vi "NGwrite_imp.vi"(0 "Unresolved URL":string, 1 "buffer value limit":u32=1, 5 "Cached URL":string, 7 "Data":variant, 9 "buffer size limit":u32=4294967295, 11 "error in":errorcluster) -> (15 "error out":errorcluster)   [LabVIEW 2017]
uses:
  nitaglv.dll
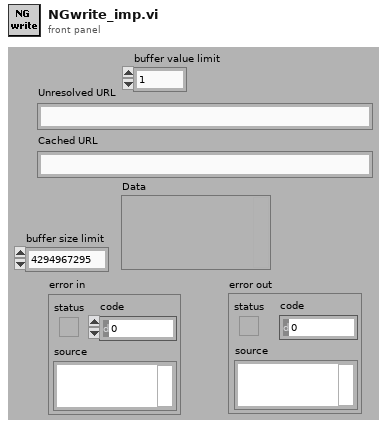
[diagram p1: front panel]
types:
  T1 = cluster{"timestamp":bool, "write":bool, "buffer size limit":u32, "buffer value limit":u32, "delta filter":bool}
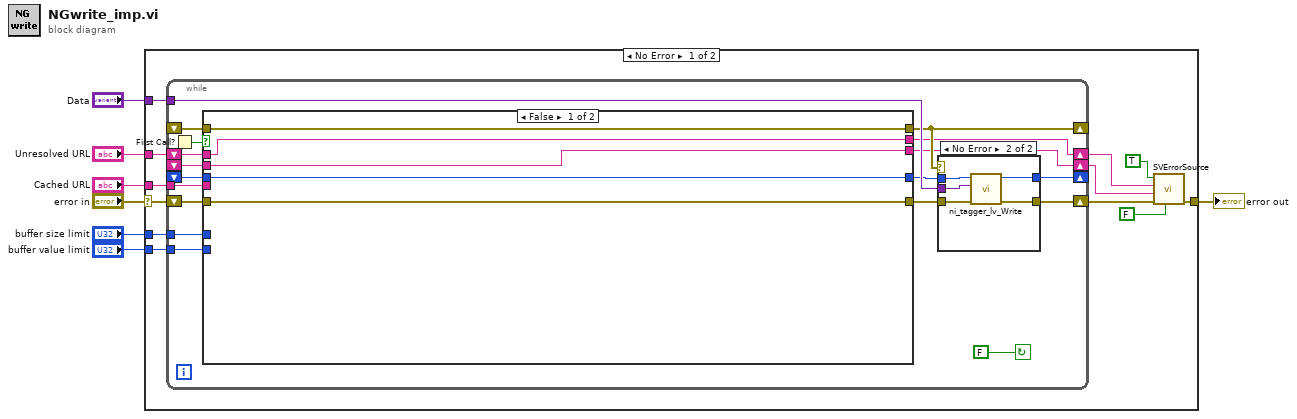
[diagram p0: block diagram]
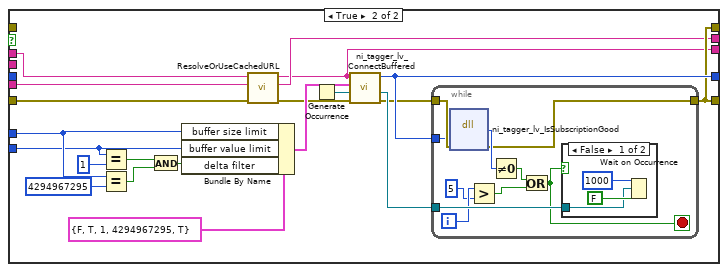
[diagram p3: hidden frame]
diagram:
  n1 = case shown="No Error" "error in" {
    selector: "error in" -> [w19 w83]
    tunnel: [w13 w83] -> w6
    tunnel: "Unresolved URL" -> [w10 _]
    tunnel: "buffer size limit" -> [w17 _]
    tunnel: "buffer value limit" -> [w16 _]
    tunnel: "Data" -> [w15 _]
    tunnel: "Cached URL" -> [w14 _]
    frame No Error {
      n2 = while {
        shift-right: [w35] -> _
        shift-left: _ -> [w33]
        tunnel: w17 -> [w29]
        tunnel: w16 -> [w28]
        tunnel: w15 -> [w27]
        tunnel: w14 -> [w26]
        shift-right: [w20] -> w8
        shift-left: _ -> [w36]
        shift-right: [w31] -> w18
        shift-left: w19 -> [w32]
        shift-right: [w23] -> _
        shift-left: _ -> [w25]
        shift-right: [w21] -> w9
        shift-left: w10 -> [w22]
        stop <- FALSE continue-if-true
        n3 = First Call?() -> (First Call?: T/F=w34:bool)
        n4 = case shown="False" w34 {
          tunnel: w36 -> [w45 _]
          tunnel: [w49 w57] -> w24
          tunnel: [w48 w53] -> w30
          tunnel: w33 -> [w49 _]
          tunnel: w32 -> [w48 w61]
          tunnel: w29 -> [_ w60]
          tunnel: w28 -> [_ w59]
          tunnel: w26 -> [_ w58]
          tunnel: [w47 w53] -> w23
          tunnel: w25 -> [w47 _]
          tunnel: w22 -> [w46 w52]
          tunnel: [w46 w51] -> w21
          tunnel: [w45 w50] -> w20
          frame False {
          }
          frame True {
            n5 = Equal?(x=w59, y=u32 1) -> (x = y?=w65:bool)
            n6 = Equal?(x=w60, y=u32 4294967295 ("buffer value limit")) -> (x = y?=w64:bool)
            n7 = And(x=w65, y=w64) -> (x .and. y?=w63:bool)
            n8 = Bundle By Name(cluster=T1 {"timestamp"=FALSE, "write"=TRUE, "buffer size limit"=1, "buffer value limit"=4294967295, "delta filter"=TRUE} ("options"), "buffer size limit"=w60, "buffer value limit"=w59, "delta filter"=w63) -> (w62:T1)
            n9 = call <vilib>:"ResolveOrUseCachedURL.vi"("error in (no error)"=w61, "Cached Resolved URL"=w58, "Unresolved URL"=w52) -> ("error out"=w55:errorcluster, "Unresolved URL out"=w51:string, "Resolved URL out"=w50:string)  [unwired: 6 in]
            n10 = Generate Occurrence() -> (w69:refnum<k4>)
            n11 = call <vilib>:"ni_tagger_lv_ConnectBuffered.vi"("error in (no error)"=w55, "read in"=w69, "options"=w62, "path"=w50) -> ("error out"=w54:errorcluster, "read out"=w56:refnum<k4>, "item"=w57:u32)  [unwired: 1 in]
            n12 = while {
              tunnel: w57 -> [w77]
              tunnel: w56 -> [w79]
              tunnel: w54 -> [w78]
              tunnel: [w75] -> w53
              i -> [w72]
              stop <- w70 stop-if-true
              n13 = dll-call lib="nitaglv.*" fn="ni_tagger_lv_IsSubscriptionGood" label="IsSubscriptionGood"("itemRefnum"=w77, "error out"=w78) -> (w76:i32, "error out"=w75:errorcluster)  [unwired: 4 in, 2 out]
              n14 = Greater?(x=w72, y=5 ("x")) -> (0:w74:bool)
              n15 = Not Equal To 0?(x=w76) -> (x != 0?=w73:bool)
              n16 = Or(x=w73, y=w74) -> (x .or. y?=w70:bool)
              n17 = case shown="False" w70 {
                tunnel: w79 -> [w80 _]
                frame False {
                  n18 = Wait on Occurrence(1:FALSE ("ignore previous (T)"), 2:w80, 3:1000 ("ms timeout (-1)")) -> ()  [unwired: 1 out]
                }
                frame True {
                }
              }
            }
          }
        }
        n19 = case shown="No Error" w23 {
          selector: w23 -> [w38 _]
          tunnel: [w39 w44] -> w35
          tunnel: [w38 w43] -> w31
          tunnel: w30 -> [_ w42]
          tunnel: w27 -> [_ w41]
          tunnel: w24 -> [w39 w40]
          frame Error {
          }
          frame No Error {
            n20 = call <vilib>:"ni_tagger_lv_Write.vi"("error in"=w42, "value"=w41, "item in"=w40) -> ("error out"=w43:errorcluster, "item out"=w44:u32)  [unwired: 3 in]
          }
        }
      }
      n21 = call <vilib>:"SVErrorSource.vi"("RT?"=FALSE, "error in"=w18, "Resolved URL"=w8, "Unresolved URL"=w9, "Write?"=TRUE) -> ("error out"=w13:errorcluster)  [unwired: 6 in]
    }
    frame Error {
    }
  }
  "error out" <- w6
